vi "Cap_Calibration.vi"(6 "INL":dbl[](array[numeric]), 7 "DNL":dbl[](array[numeric]), 8 "From File/ Waveform":bool, 9 "Select Channel":enum16{"Even Channel", "Odd Channel"}(ring), 10 "Average Window":dbl=8.0, 11 "File path (DNL & INL)":path) -> (1 "ADC TEST 7":string, 2 "ADC TEST 6":string, 3 "ADC TEST 5":string, 4 "Trim Coeff (Binary)":string[](array[string]), 5 "Trim Coeff (Integer)":dbl[](array[numeric]))   [LabVIEW 2021]
doc: "Calculateds Capcitor mismatch from the INL/DNL."
uses:
  <vilib>/Utility/file.llb/Read From Spreadsheet File (DBL).vi
panel:
  out "Trim Coeff (real)":dbl[](array[numeric]) format="%#_9g"
  out "Scaled":dbl[](array[numeric])
  out "INL Jumps":dbl[](array[numeric])
  out "INL Jump":dbl[](array[numeric])
  out "all rows":dbl[][](array[numeric]) format="%0.4f"
  out "Center Code":i32[](array[numeric])
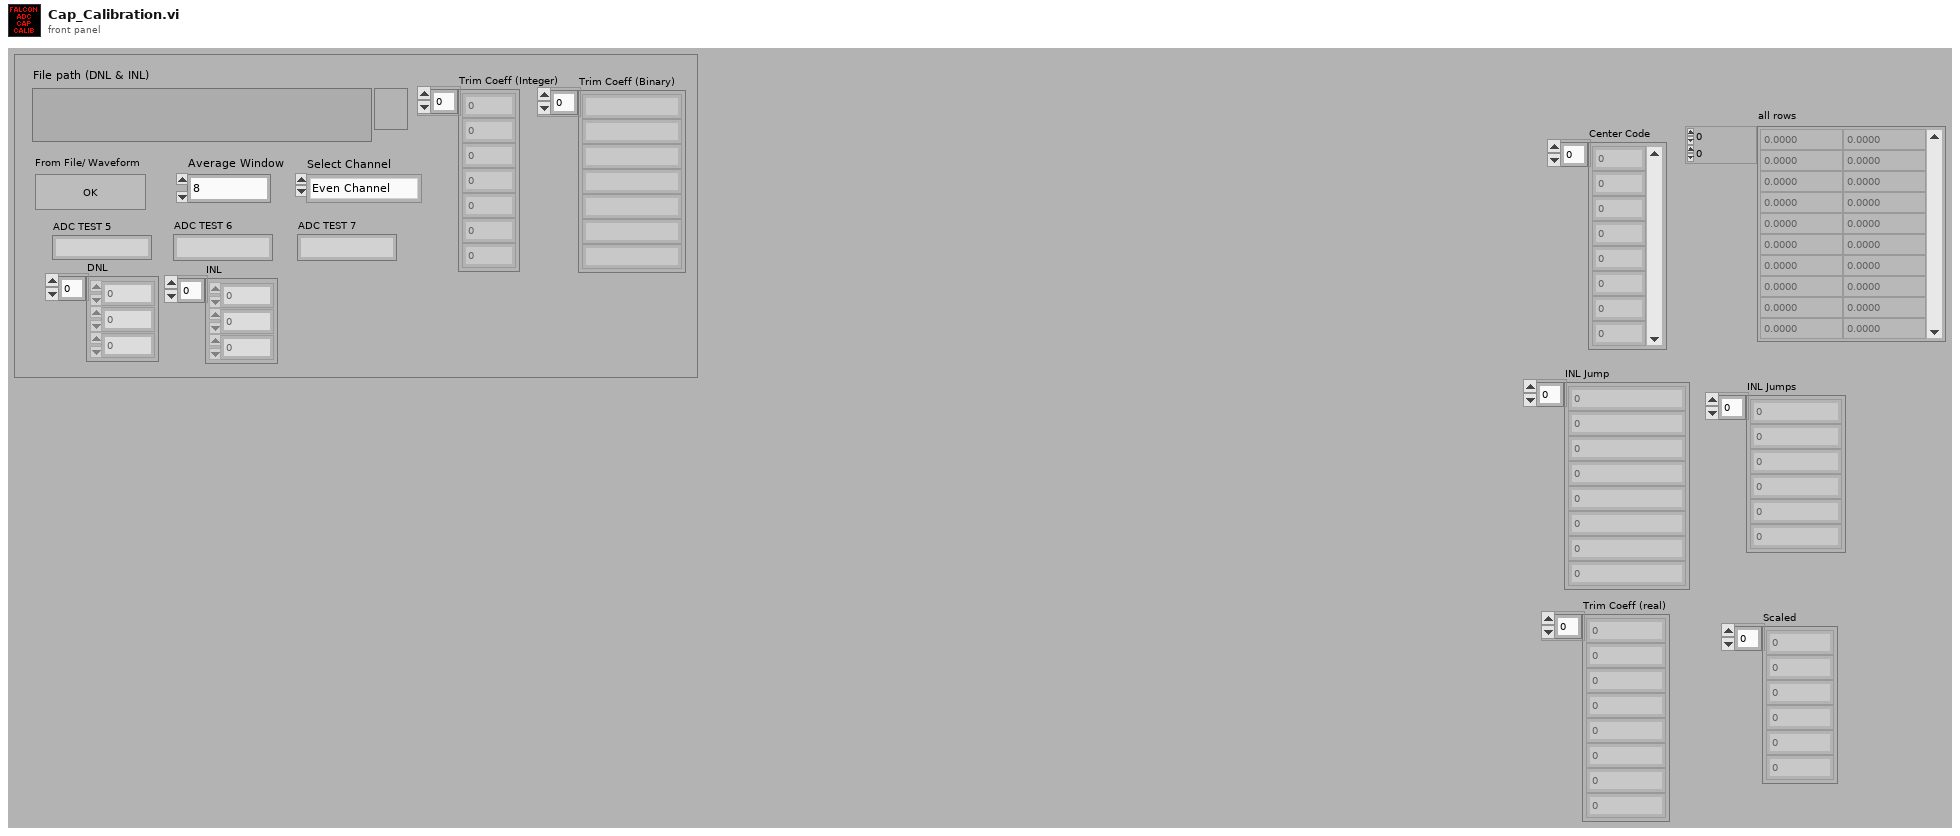
[diagram p1: front panel]
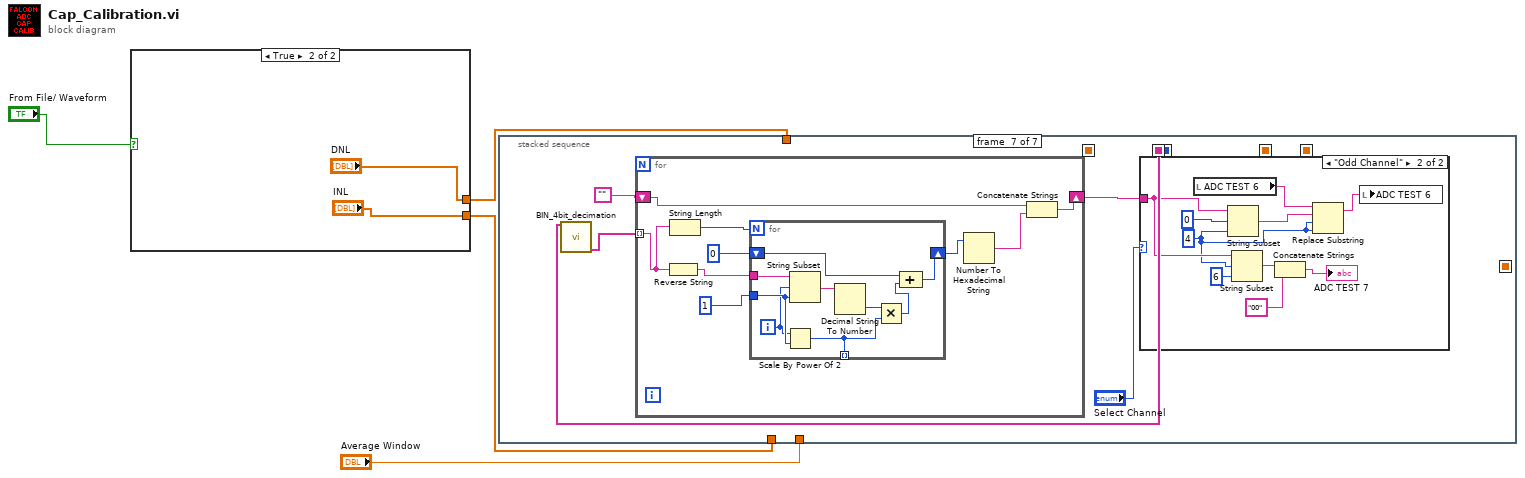
[diagram p0: block diagram]
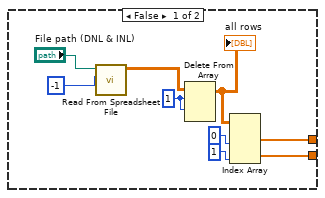
[diagram p2: hidden frame]
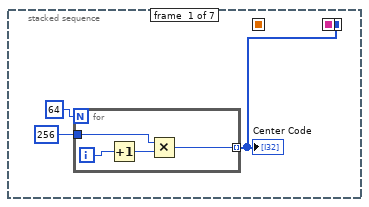
[diagram p3: hidden frame]
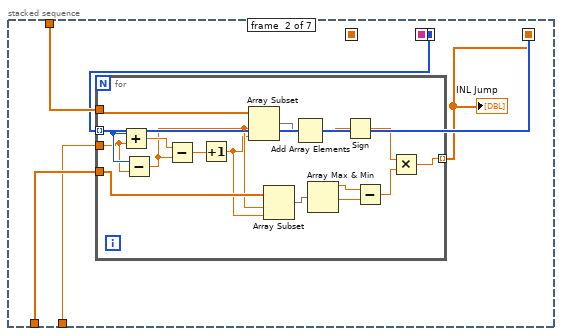
[diagram p4: hidden frame]
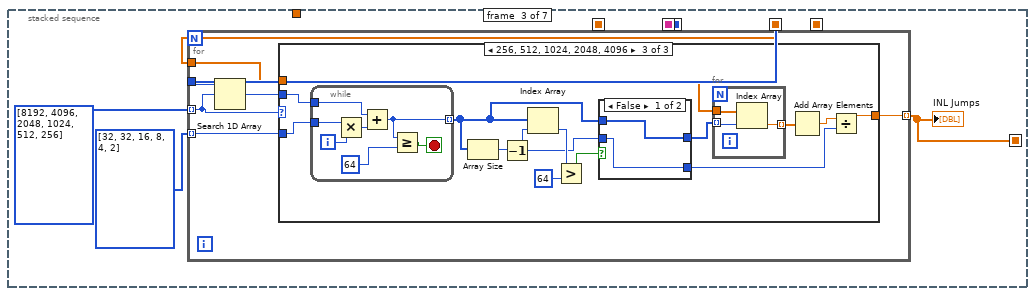
[diagram p5: hidden frame]
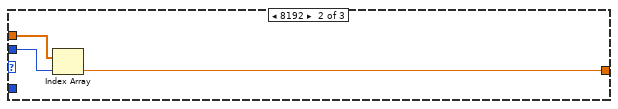
[diagram p7: hidden frame]
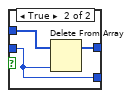
[diagram p8: hidden frame]
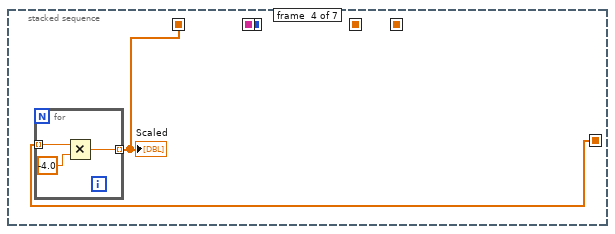
[diagram p9: hidden frame]
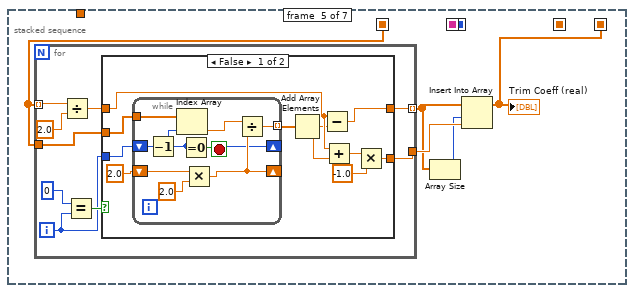
[diagram p10: hidden frame]
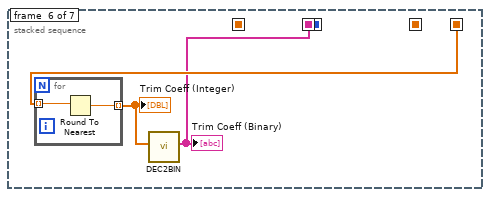
[diagram p12: hidden frame]
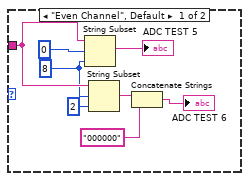
[diagram p13: hidden frame]
diagram:
  n1 = case shown="True" "From File/ Waveform" {
    tunnel: [w6 "DNL"] -> w4
    tunnel: [w5 "INL"] -> w3
    frame False {
      w10 = 1 ("length")
      n2 = call-poly <vilib>:"Read From Spreadsheet File.vi"("number of rows (all:-1)"=-1, "file path (dialog if empty)"="File path (DNL & INL)") -> ("all rows"=w11:dbl[][])  [unwired: 5 in, 4 out]
      n3 = Delete From Array(array=w11, length=w10, index (row)=w10) -> (array with subset deleted=w9:dbl[][])  [unwired: 1 in, 1 out]
      "all rows" <- w9
      n4 = Index Array(array=w9, index (col) #1=0 ("index (row)"), index (col) #2=1 ("index (row)")) -> (element #1=w6:dbl[], element #2=w5:dbl[])  [unwired: 2 in]
    }
    frame True {
    }
  }
  n5 = stacked-sequence {
    seq-local: [w16 _ _ _ _ _ _] -> [_ w24 _ _ _ _ _]
    seq-local: [_ w24 _ _ _ _ _] -> [_ _ w47 _ _ _ _]
    seq-local: [_ w23 _ _ _ _ _] -> [_ _ w46 _ _ _ _]
    seq-local: [_ _ w44 _ _ _ _] -> [_ _ _ w88 _ _ _]
    seq-local: [_ _ _ w87 _ _ _] -> [_ _ _ _ w96 _ _]
    seq-local: [_ _ _ _ w92 _ _] -> [_ _ _ _ _ w128 _]
    seq-local: [_ _ _ _ _ w126 _] -> [_ _ _ _ _ _ w135]
    tunnel: w4 -> [_ w27 _ _ _ _ _]
    tunnel: w3 -> [_ w26 _ _ _ _ _]
    tunnel: "Average Window" -> [_ w25 _ _ _ _ _]
    frame #0 {
      n6 = for {
        N: 64 -> [_]
        tunnel: 256 -> [w20]
        tunnel: [w19] -> w16 mode=indexing
        i -> [w22]
        n7 = Increment(x=w22) -> (x+1=w21:i32)
        n8 = Multiply(x=w20, y=w21) -> (x*y=w19:i32)
      }
      "Center Code" <- w16
    }
    frame #1 {
      n9 = for {
        tunnel: w24 -> [w43] mode=indexing
        tunnel: w27 -> [w41]
        tunnel: w26 -> [w37]
        tunnel: w25 -> [w42]
        tunnel: [w29] -> w23 mode=indexing
        n10 = Add(x=w43, y=w42) -> (x+y=w39:dbl)
        n11 = Subtract(x=w43, y=w42) -> (x-y=w36:dbl)
        n12 = Subtract(x=w39, y=w36) -> (x-y=w40:dbl)
        n13 = Increment(x=w40) -> (x+1=w35:dbl)
        n14 = Array Subset(array=w41, index=w36, length=w35) -> (w38:dbl[])
        n15 = Array Subset(array=w37, index=w36, length=w35) -> (w34:dbl[])
        n16 = Add Array Elements(numeric array=w38) -> (sum=w30:dbl)
        n17 = Array Max & Min(array=w34) -> (max value=w33:dbl, min value=w32:dbl)  [unwired: 2 out]
        n18 = Sign(1:w30) -> (0:w28:dbl)
        n19 = Subtract(x=w33, y=w32) -> (x-y=w31:dbl)
        n20 = Multiply(x=w28, y=w31) -> (x*y=w29:dbl)
      }
      "INL Jump" <- w23
    }
    frame #2 {
      n21 = for {
        tunnel: i32[] [8192, 4096, 2048, 1024, 512, 256] -> [w52] mode=indexing
        tunnel: w47 -> [w54]
        tunnel: w46 -> [w51]
        tunnel: [w53] -> w44 mode=indexing
        tunnel: i32[] [32, 32, 16, 8, 4, 2] -> [w49] mode=indexing
        n22 = Search 1D Array(1D array=w54, element=w52) -> (index of element=w50:i32)  [unwired: 1 in]
        n23 = case shown="256, 512, 1024, 2048, 4096" w52 {
          tunnel: [_ w55 w66] -> w53
          tunnel: w51 -> [_ w57 w69]
          tunnel: w50 -> [_ w56 w71]
          tunnel: w49 -> [_ _ w70]
          frame 0, Default {
          }
          frame 8192 {
            n24 = Index Array(array=w57, index=w56) -> (element=w55:dbl)
          }
          frame 256, 512, 1024, 2048, 4096 {
            n25 = while {
              tunnel: w71 -> [w83]
              tunnel: w70 -> [w86]
              tunnel: [w81] -> w62 mode=indexing
              i -> [w85]
              stop <- w82 stop-if-true
              n26 = Multiply(x=w86, y=w85) -> (x*y=w84:i32)
              n27 = Add(x=w83, y=w84) -> (x+y=w81:i32)
              n28 = Greater Or Equal?(x=w81, y=64) -> (x >= y?=w82:bool)
            }
            n29 = Array Size(array=w62) -> (size(s)=w58:i32)
            n30 = Decrement(x=w58) -> (x-1=w61:i32)
            n31 = Index Array(array=w62, index=w61) -> (element=w65:i32)
            n32 = Greater?(x=w65, y=64) -> (0:w63:bool)
            n33 = case shown="False" w63 {
              tunnel: w62 -> [w73 w76]
              tunnel: w61 -> [w72 w74]
              tunnel: [w73 w75] -> w60
              tunnel: [w72 w74] -> w59
              frame False {
              }
              frame True {
                n34 = Delete From Array(array=w76, index=w74) -> (array with subset deleted=w75:i32[])  [unwired: 1 in, 1 out]
              }
            }
            n35 = for {
              tunnel: w60 -> [w78] mode=indexing
              tunnel: w69 -> [w79]
              tunnel: [w77] -> w68 mode=indexing
              n36 = Index Array(array=w79, index=w78) -> (element=w77:dbl)
            }
            n37 = Add Array Elements(numeric array=w68) -> (sum=w67:dbl)
            n38 = Divide(x=w67, y=w59) -> (x/y=w66:dbl)
          }
        }
      }
      "INL Jumps" <- w44
    }
    frame #3 {
      n39 = for {
        tunnel: w88 -> [w91] mode=indexing
        tunnel: [w89] -> w87 mode=indexing
        n40 = Multiply(x=w91, y=-4.0) -> (x*y=w89:dbl)
      }
      "Scaled" <- w87
    }
    frame #4 {
      n41 = for {
        tunnel: w96 -> [w105] mode=indexing
        tunnel: [w100] -> w94 mode=indexing
        tunnel: w96 -> [w99]
        tunnel: [w97] -> w95
        i -> [w98]
        n42 = Divide(x=w105, y=2.0) -> (x/y=w101:dbl)
        n43 = Equal?(x=0, y=w98) -> (x = y?=w102:bool)
        n44 = case shown="False" w102 {
          tunnel: w101 -> [w110 w125]
          tunnel: [w111 w125] -> w100
          tunnel: w99 -> [w115 _]
          tunnel: w98 -> [w114 _]
          tunnel: [w107 _] -> w97
          frame False {
            n45 = while {
              tunnel: w115 -> [w124]
              shift-right: [w119] -> _
              shift-left: 2.0 ("y") -> [w121]
              tunnel: [w117] -> w112 mode=indexing
              shift-right: [w116] -> _
              shift-left: w114 -> [w123]
              stop <- w122 stop-if-true
              n46 = Decrement(x=w123) -> (x-1=w116:i32)
              n47 = Index Array(array=w124, index=w116) -> (element=w118:dbl)
              n48 = Equal To 0?(x=w116) -> (x = 0?=w122:bool)
              n49 = Multiply(x=w121, y=2.0) -> (x*y=w119:dbl)
              n50 = Divide(x=w118, y=w119) -> (x/y=w117:dbl)
            }
            n51 = Add Array Elements(numeric array=w112) -> (sum=w109:dbl)
            n52 = Subtract(x=w110, y=w109) -> (x-y=w111:dbl)
            n53 = Add(x=w110, y=w109) -> (x+y=w108:dbl)
            n54 = Multiply(x=w108, y=-1.0) -> (x*y=w107:dbl)
          }
          frame True {
          }
        }
      }
      n55 = Array Size(array=w94) -> (size(s)=w93:i32)
      n56 = Insert Into Array(array=w94, index=w93, new element=w95) -> (w92:dbl[])
      "Trim Coeff (real)" <- w92
    }
    frame #5 {
      n57 = for {
        tunnel: w128 -> [w130] mode=indexing
        tunnel: [w129] -> w127 mode=indexing
        n58 = Round To Nearest(number=w130) -> (nearest integer value=w129:dbl)
      }
      "Trim Coeff (Integer)" <- w127
      n59 = call "DEC2BIN.vi"("DECIMAL"=w127) -> ("BINARY"=w126:string[])  [unwired: 10 in]
      "Trim Coeff (Binary)" <- w126
    }
    frame #6 {
      n60 = call "BIN_4bit_decimation.vi"("BINARY"=w135) -> ("Array"=w134:string[])  [unwired: 3 in, 11 out]
      n61 = for {
        tunnel: w134 -> [w158] mode=indexing
        shift-right: [w154] -> w132
        shift-left: "" -> [w156]
        n62 = Reverse String(1:w158) -> (0:w159:string)
        n63 = String Length(string=w158) -> (length=w160:i32)
        n64 = for {
          N: w160 -> [_]
          tunnel: w159 -> [w171]
          tunnel: 1 ("offset (0)") -> [w167]
          shift-right: [w165] -> w157
          shift-left: 0 ("offset (0)") -> [w164]
          tunnel: [w163] -> _ mode=indexing
          i -> [w166]
          n65 = Scale By Power Of 2(n=w166, x=w167) -> (x*2^n=w163:i32)
          n66 = String Subset(string=w171, offset (0)=w166, length (rest)=w167) -> (substring=w170:string)
          n67 = Decimal String To Number(string=w170) -> (number=w169:i32)  [unwired: 2 in, 1 out]
          n68 = Multiply(x=w169, y=w163) -> (x*y=w168:i32)
          n69 = Compound Arithmetic op=ADD(w164, w168) -> (w165:i32)
        }
        n70 = Number To Hexadecimal String(2:w157) -> (0:w155:string)  [unwired: 1 in]
        n71 = Concatenate Strings(w156, w155) -> (w154:string)
      }
      n72 = case shown="\"Odd Channel\"" "Select Channel" {
        tunnel: w132 -> [w141 w152]
        frame "Even Channel", Default {
          w140 = 8 ("length (rest)")
          n73 = String Subset(string=w141, offset (0)=0, length (rest)=w140) -> (substring=→"ADC TEST 5":string)
          n74 = String Subset(string=w141, offset (0)=w140, length (rest)=2 ("length (rest)")) -> (substring=w138:string)
          n75 = Concatenate Strings(w138, "000000" ("string")) -> (→"ADC TEST 6":string)
        }
        frame "Odd Channel" {
          w145 = 4 ("length (rest)")
          n76 = local read "ADC TEST 6"() -> (w147:string)
          n77 = String Subset(string=w152, offset (0)=0, length (rest)=w145) -> (substring=w146:string)
          n78 = String Subset(string=w152, offset (0)=w145, length (rest)=6 ("length (rest)")) -> (substring=w150:string)
          n79 = Concatenate Strings(w150, "00" ("string")) -> (→"ADC TEST 7":string)
          n80 = Replace Substring(2:w145, 3:w145, 4:w146, 5:w147) -> (1:w144:string)  [unwired: 1 out]
          n81 = local write "ADC TEST 6"(w144) -> ()
        }
      }
    }
  }
